vi "Untitled 1.vi"() -> ()   [LabVIEW 2020]
panel:
  out "Resitência termica":bool
  out "Ventoinha":bool
  out "Temperatura ºC":dbl
  out "Temperatura  ºC":dbl(graph)
  in  "Temperatura desejada ºC":dbl min=0.0 max=50.0 step=0.01 format="%#_6f"
  out "Ccs1":bool
  out "Tempo de funcionamento":dbl
  out "Temperatura Máxima ºC":dbl
  out "Temperatura Mínima ºC":dbl
  in  "reset":bool
  out "Temperatura ºC":dbl
  out "Temperatura °F":dbl
  out "Temperatura K":dbl
  out "Saida do AI":dbl
  out "Condicionamento de sinal 2":dbl
  out "Condicionamento de sinal 1":dbl
  out "Ccs2":bool
  in  "stop":bool
  in  "Temperatura":ext(slide) caption="Thermometer" scale=0.0..50.0
  in  "Limite inferior":dbl step=0.001
  in  "Limite superior":dbl step=0.001
  in  "Valor de referencia":dbl step=0.1
  out "Condicionamento de sinal 2":dbl(graph)
  out "Condicionamento de sinal 1":dbl(graph)
  in  "Tensão de alimentação":dbl
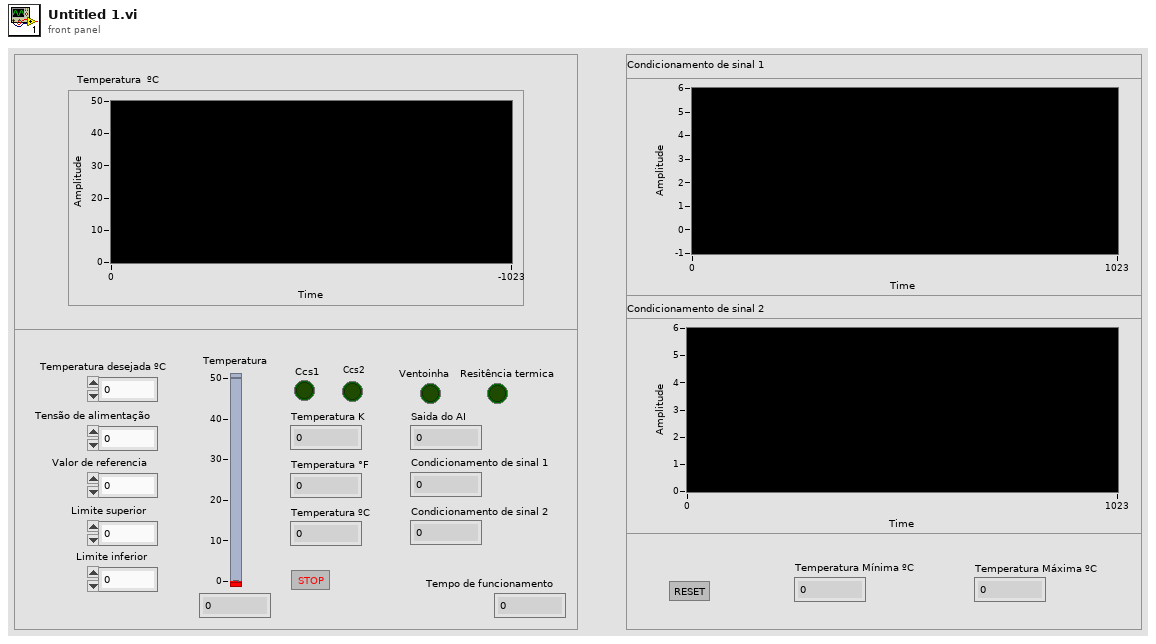
[diagram p1: front panel]
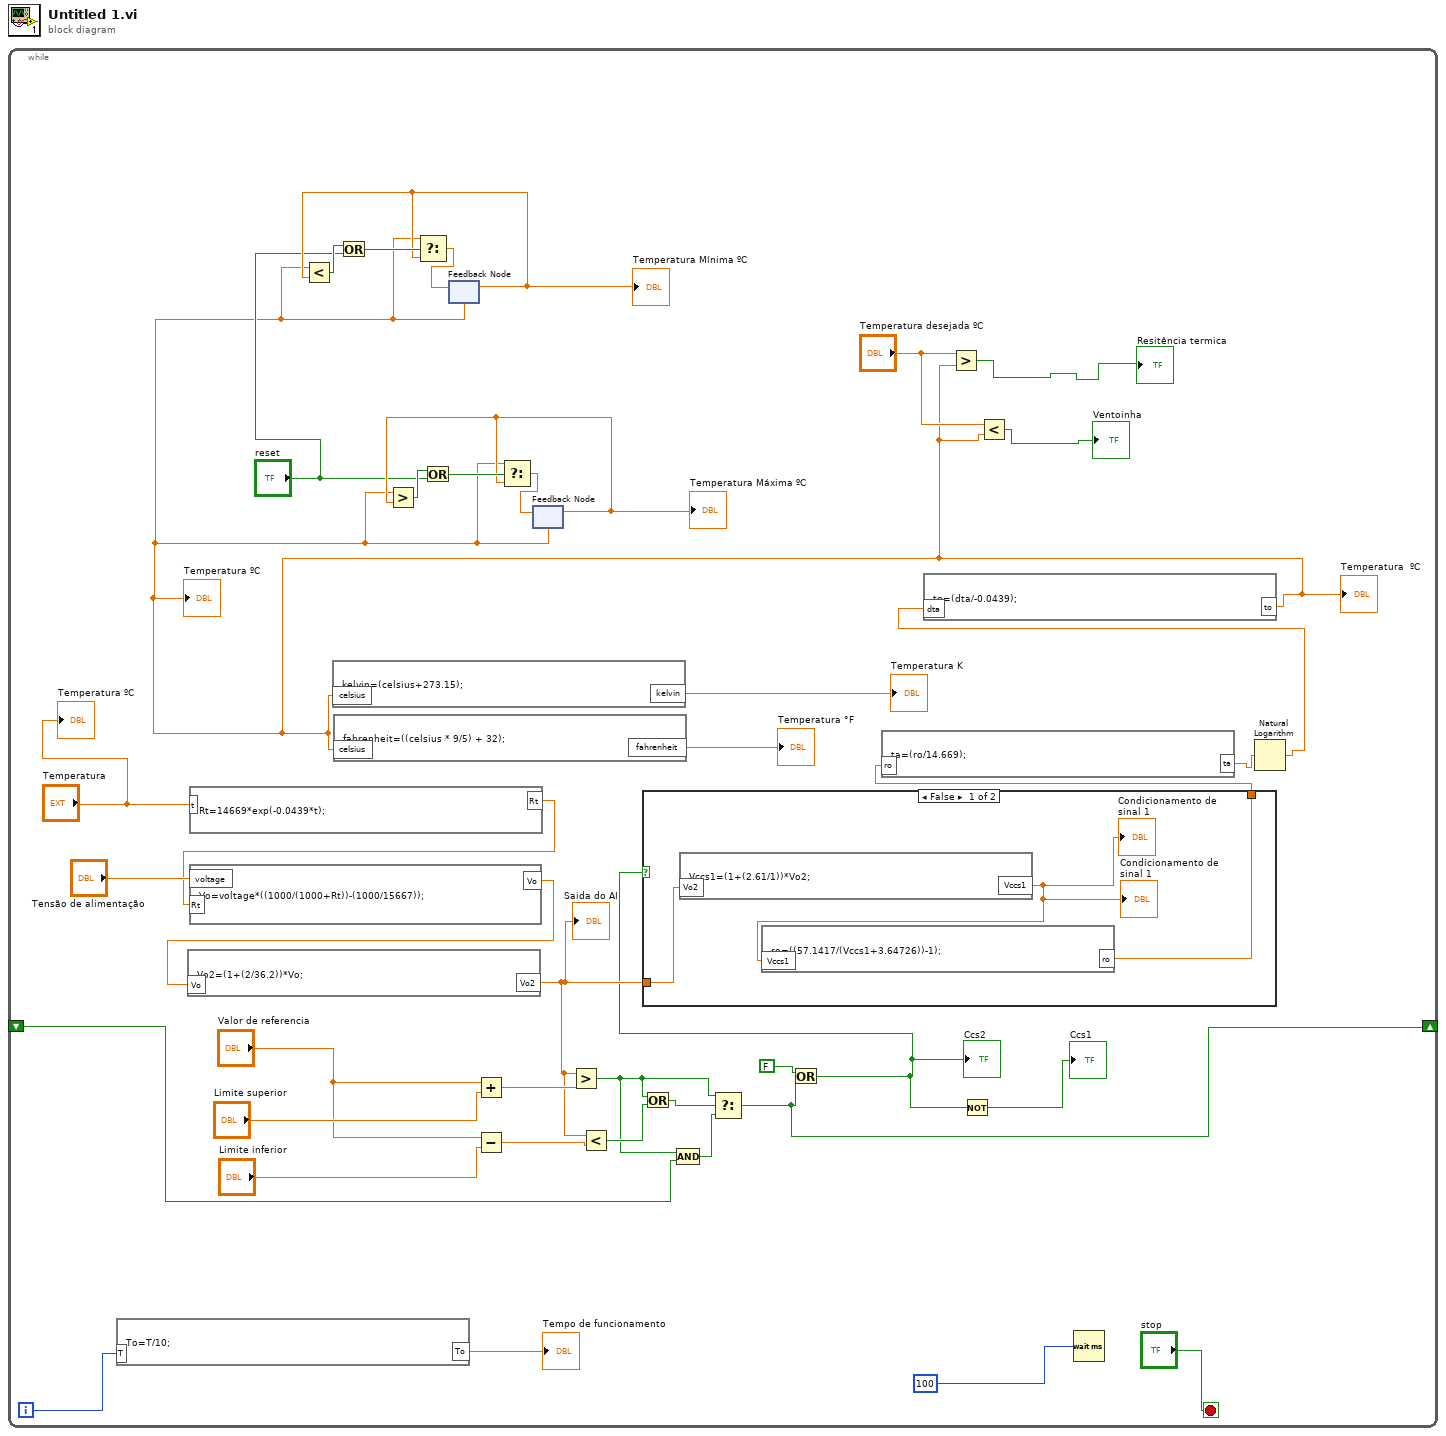
[diagram p0: block diagram]
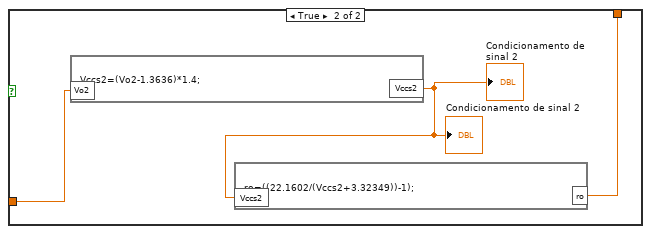
[diagram p2: hidden frame]
diagram:
  n1 = while {
    shift-right: [w28] -> _
    shift-left: _ -> [w29]
    i -> [w15]
    stop <- "stop" stop-if-true
    n2 = formula code="To=T/10;"("T"=w15) -> ("To"=→"Tempo de funcionamento":dbl)
    n3 = formula code="Rt=14669*exp(-0.0439*t);"("t"="Temperatura") -> ("Rt"=w40:dbl)
    n4 = formula code="Vo=voltage*((1000/(1000+Rt))-(1000/15667));"("voltage"="Tensão de alimentação", "Rt"=w40) -> ("Vo"=w39:dbl)
    n5 = formula code="Vo2=(1+(2/36.2))*Vo;"("Vo"=w39) -> ("Vo2"=w24:dbl)
    "Saida do AI" <- w24
    n6 = Add(x="Valor de referencia", y="Limite superior") -> (x+y=w35:dbl)
    n7 = Subtract(x="Valor de referencia", y="Limite inferior") -> (x-y=w34:dbl)
    n8 = Greater?(x=w24, y=w35) -> (0:w30:bool)
    n9 = Less?(x=w24, y=w34) -> (x < y?=w33:bool)
    n10 = Or(x=w30, y=w33) -> (x .or. y?=w32:bool)
    n11 = Compound Arithmetic op=AND(w30, w29) -> (w27:bool)
    n12 = Select(t=w30, s=w32, f=w27) -> (s? t:f=w28:bool)
    n13 = Or(x=FALSE, y=w28) -> (x .or. y?=w10:bool)
    "Ccs2" <- w10
    n14 = case shown="False" w10 {
      tunnel: w24 -> [w44 w47]
      tunnel: [w42 w45] -> w8
      frame False {
        n15 = formula code="Vccs1=(1+(2.61/1))*Vo2;"("Vo2"=w44) -> ("Vccs1"=w43:dbl)
        "Condicionamento de sinal 1" <- w43
        "Condicionamento de sinal 1" <- w43
        n16 = formula code="ro=((57.1417/(Vccs1+3.64726))-1);"("Vccs1"=w43) -> ("ro"=w42:dbl)
      }
      frame True {
        n17 = formula code="Vccs2=(Vo2-1.3636)*1.4;"("Vo2"=w47) -> ("Vccs2"=w46:dbl)
        "Condicionamento de sinal 2" <- w46
        "Condicionamento de sinal 2" <- w46
        n18 = formula code="ro=((22.1602/(Vccs2+3.32349))-1);"("Vccs2"=w46) -> ("ro"=w45:dbl)
      }
    }
    n19 = formula code="ta=(ro/14.669);"("ro"=w8) -> ("ta"=w7:dbl)
    n20 = Not(x=w10) -> (.not. x?=→"Ccs1":bool)
    n21 = Wait (ms)(milliseconds to wait=100) -> ()  [unwired: 1 out]
    n22 = Natural Logarithm(1:w7) -> (0:w6:dbl)
    n23 = formula code="to=(dta/-0.0439);"("dta"=w6) -> ("to"=w3:dbl)
    "Temperatura ºC" <- w3
    "Temperatura  ºC" <- w3
    n24 = formula code="kelvin=(celsius+273.15);"("celsius"=w3) -> ("kelvin"=→"Temperatura K":dbl)
    n25 = formula code="fahrenheit=((celsius * 9/5) + 32);"("celsius"=w3) -> ("fahrenheit"=→"Temperatura °F":dbl)
    n26 = feedback #1(w3) -> (w16:dbl)
    "Temperatura Mínima ºC" <- w16
    n27 = Less?(x=w3, y=w16) -> (x < y?=w18:bool)
    n28 = Or(x=w18, y="reset") -> (x .or. y?=w17:bool)
    n29 = Select(t=w3, s=w17, f=w16) -> (s? t:f=w11:dbl)
    n30 = feedback-in #1(w11) -> ()
    n31 = feedback #2(w3) -> (w19:dbl)
    "Temperatura Máxima ºC" <- w19
    n32 = Greater?(x=w3, y=w19) -> (0:w21:bool)
    n33 = Or(x=w21, y="reset") -> (x .or. y?=w20:bool)
    n34 = Select(t=w3, s=w20, f=w19) -> (s? t:f=w12:dbl)
    n35 = feedback-in #2(w12) -> ()
    n36 = Greater?(x="Temperatura desejada ºC", y=w3) -> (0:→"Resitência termica":bool)
    n37 = Less?(x="Temperatura desejada ºC", y=w3) -> (x < y?=→"Ventoinha":bool)
    "Temperatura ºC" <- "Temperatura"
  }
